vi "Virtual Labs 3.0.11.vi"() -> ()   [LabVIEW 2014]
panel:
  out "Actual volt":dbl
  out "Actual level":i32
  out "Ideal Vevel":i32
  out "Ideal voltage":dbl
  out "Stop":bool
  in  "Tab Control":T1(tab)
  in  "2":dbl(slide) scale=0.0..25.0
  out "?":dbl format="%#_3g"
  out "?":dbl format="%#_3g"
  out "?":dbl(slide) scale=0.0..684.0
  out "?":bool
  in  "Master Stop 2":bool
  out "Table 2":string[][](table)
  in  "Potentiometer\n       (4.7K)":dbl(knob) scale=0.0..4700.0 scale format="%#_6p"
  in  "Potentiometer (10K)":dbl(knob) scale=0.0..10000.0 scale format="%#_6p"
  out "?":dbl(slide) scale=0.0..684.0
  out "?":dbl format="%#_3g"
  out "?":dbl format="%#_3g"
  in  "?":dbl(slide)=25.0 scale=0.0..25.0
  out "?":bool
  in  "Master Stop":bool
  out "Table 3":string[][](table)
  out "Level Vs Output Voltage":cluster{"Y":dbl[], "Y":dbl[]}[](graph)
  out "Table 4":string[][](table)
  # "Manipal Institute of Technology  \n        Dept of Instrumentation and Control Engineering\n                                 V Sem (Instrumentation Lab)"
  # "VIRTUAL LABS"
  # "VIRTUAL LABS"
  # "EXPERIMENT NO.1"
  # "Liquid Level Measurement Using Capacitance Level Sensor\n\nObjective:  To design a signal conditioning circuit for measurement of liquid level using capacitance level sensors. \n\nApparatus required:\n\n            1\tCLS\n            2\tResistances\n            3\tAmplifier (741)\n            4\tDC power supply\n            5\tDMM"
  # "Ideal Case"
  # "Capacitive Level Sensor"
  # "Digital Multimeter"
  # "4-20m A"
  # "Level (in mm)"
  # "DC Voltage\n        (V)"
  # "Current (mA)"
  # "Animation Speed"
  # "Master Stop"
  # "Capacitive Level Sensor"
  # "Digital Multimeter"
  # "4-20m A"
  # "Level (in mm)"
  # "DC Voltage\n        (V)"
  # "Current (mA)"
  # "Animation Speed"
  # "Master Stop"
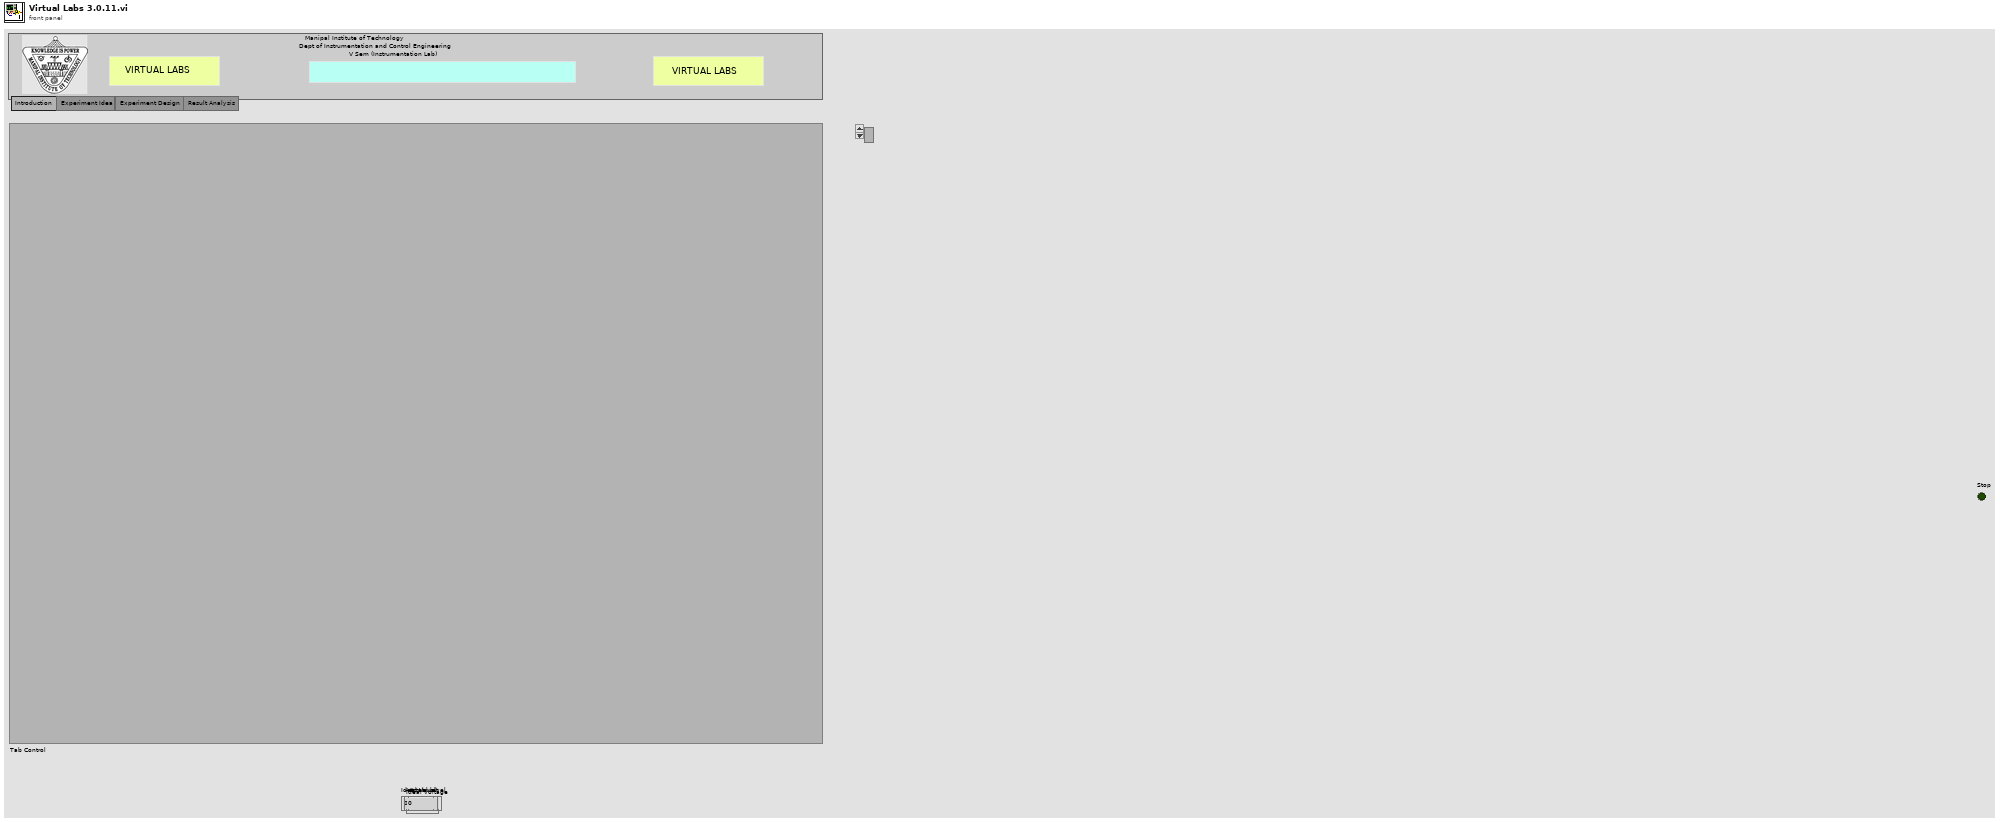
[diagram p1: front panel]
types:
  T1 = enum32{"Introduction", "Experiment Idea", "Experiment Design ", "Result Analysis"}
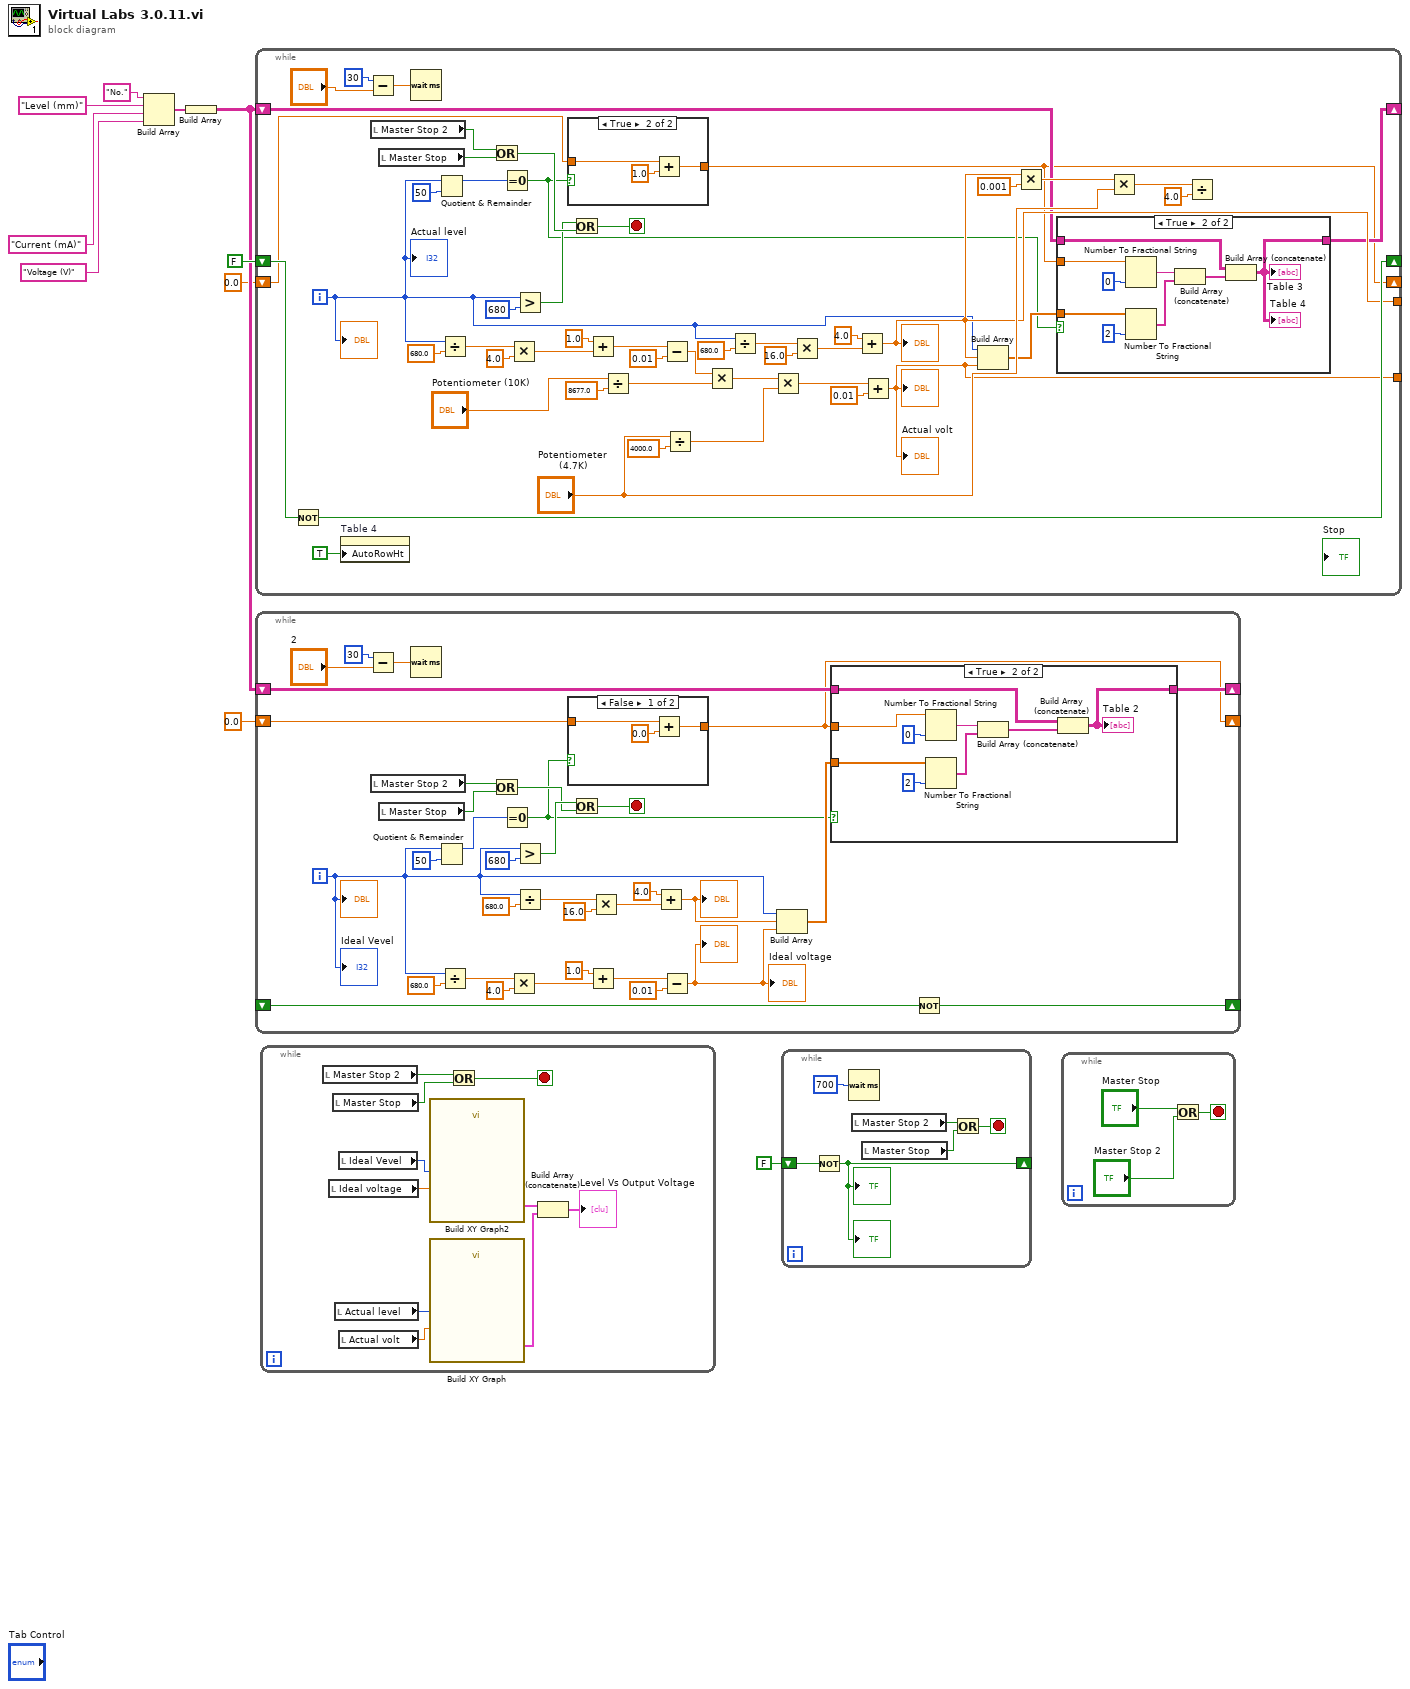
[diagram p0: block diagram]
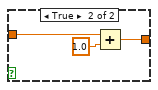
[diagram p2: hidden frame]
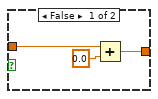
[diagram p4: hidden frame]
diagram:
  n1 = Build Array("No." ("element"), "Level (mm)" ("element"), "Current (mA)", "Voltage (V)") -> (w7:string[])
  n2 = Build Array(w7) -> (w6:string[][])
  n3 = while {
    shift-right: [w45] -> _
    shift-left: FALSE -> [w46]
    tunnel: [w14] -> _
    tunnel: [w25] -> _
    shift-right: [w24] -> _
    shift-left: w6 -> [w23]
    shift-right: [w11] -> _
    shift-left: 0.0 -> [w13]
    i -> [w15]
    stop <- w27 stop-if-true
    n4 = Not(x=w46) -> (.not. x?=w45:bool)
    n5 = property on="Table 4" class="Tbl (strict)"("AutoRowHt"=TRUE ("Autosizing Row Height")) -> ()  [unwired: 2 in, 2 out]
    n6 = Subtract(x=u32 30 ("milliseconds to wait"), y="?") -> (x-y=w34:dbl)
    n7 = local read "Master Stop 2"() -> (w21:bool)
    n8 = local read "Master Stop"() -> (w20:bool)
    n9 = Wait (ms)(milliseconds to wait=w34) -> ()  [unwired: 1 out]
    n10 = Quotient & Remainder(x=w15, y=50) -> (x-y*floor(x/y)=w16:i32)  [unwired: 1 out]
    n11 = Divide(x=w15, y=680.0) -> (x/y=w56:dbl)
    n12 = Or(x=w21, y=w20) -> (x .or. y?=w19:bool)
    n13 = Equal To 0?(x=w16) -> (x = 0?=w12:bool)
    n14 = Multiply(x=w56, y=4.0) -> (x*y=w54:dbl)
    n15 = Greater?(x=w15, y=680) -> (0:w18:bool)
    n16 = case shown="True" w12 {
      tunnel: w13 -> [w61 w65]
      tunnel: [w60 w64] -> w11
      frame False {
        n17 = Add(x=w61, y=0.0) -> (x+y=w60:dbl)
      }
      frame True {
        n18 = Add(x=w65, y=1.0) -> (x+y=w64:dbl)
      }
    }
    n19 = Or(x=w18, y=w19) -> (x .or. y?=w27:bool)
    n20 = Add(x=1.0, y=w54) -> (x+y=w48:dbl)
    n21 = Divide(x="Potentiometer (10K)", y=8677.0) -> (x/y=w38:dbl)
    n22 = Subtract(x=w48, y=0.01) -> (x-y=w37:dbl)
    n23 = Divide(x="Potentiometer\n       (4.7K)", y=4000.0) -> (x/y=w30:dbl)
    n24 = Multiply(x=w37, y=w38) -> (x*y=w31:dbl)
    n25 = Divide(x=w15, y=680.0) -> (x/y=w51:dbl)
    n26 = Multiply(x=w31, y=w30) -> (x*y=w29:dbl)
    n27 = Multiply(x=w51, y=16.0) -> (x*y=w53:dbl)
    n28 = Add(x=4.0, y=w53) -> (x+y=w25:dbl)
    "?" <- w25
    n29 = Add(x=w29, y=0.01) -> (x+y=w14:dbl)
    "?" <- w14
    "Actual volt" <- w14
    n30 = Build Array(w15, w25, w14) -> (w26:dbl[])
    n31 = Multiply(x=w25, y=0.001) -> (x*y=w43:dbl)
    n32 = case shown="True" w12 {
      tunnel: w26 -> [_ w75]
      tunnel: [w66 w67] -> w24
      tunnel: w23 -> [w66 w74]
      tunnel: w11 -> [_ w68]
      frame False {
      }
      frame True {
        n33 = Number To Fractional String(number=w68, precision (6)=i16 0) -> (F-format string=w71:string)  [unwired: 2 in]
        n34 = Number To Fractional String(number=w75, precision (6)=i16 2) -> (F-format string=w70:string[])  [unwired: 2 in]
        n35 = Build Array (concatenate)(w71, w70) -> (w69:string[])
        n36 = Build Array (concatenate)(w74, w69) -> (w67:string[][])
        "Table 3" <- w67
        "Table 4" <- w67
      }
    }
    n37 = Multiply(x=w43, y="Potentiometer\n       (4.7K)") -> (x*y=w42:dbl)
    n38 = Divide(x=w42, y=4.0) -> ()  [unwired: 1 out]
    "?" <- w15
    "Actual level" <- w15
  }
  n39 = while {
    shift-right: [w95] -> _
    shift-left: _ -> [w96]
    shift-right: [w86] -> _
    shift-left: w6 -> [w88]
    shift-right: [w76] -> _
    shift-left: 0.0 -> [w77]
    i -> [w83]
    stop <- w90 stop-if-true
    n40 = Subtract(x=u32 30 ("milliseconds to wait"), y="2") -> (x-y=w92:dbl)
    n41 = local read "Master Stop 2"() -> (w81:bool)
    n42 = local read "Master Stop"() -> (w80:bool)
    n43 = Wait (ms)(milliseconds to wait=w92) -> ()  [unwired: 1 out]
    n44 = Quotient & Remainder(x=w83, y=50) -> (x-y*floor(x/y)=w84:i32)  [unwired: 1 out]
    n45 = Divide(x=w83, y=680.0) -> (x/y=w106:dbl)
    n46 = Or(x=w81, y=w80) -> (x .or. y?=w79:bool)
    n47 = Equal To 0?(x=w84) -> (x = 0?=w78:bool)
    n48 = Multiply(x=w106, y=4.0) -> (x*y=w104:dbl)
    n49 = Greater?(x=w83, y=680) -> (0:w91:bool)
    n50 = Divide(x=w83, y=680.0) -> (x/y=w101:dbl)
    n51 = case shown="False" w78 {
      tunnel: w77 -> [w111 w115]
      tunnel: [w110 w114] -> w76
      frame False {
        n52 = Add(x=w111, y=0.0) -> (x+y=w110:dbl)
      }
      frame True {
        n53 = Add(x=w115, y=1.0) -> (x+y=w114:dbl)
      }
    }
    n54 = Or(x=w91, y=w79) -> (x .or. y?=w90:bool)
    n55 = Add(x=1.0, y=w104) -> (x+y=w98:dbl)
    n56 = Multiply(x=w101, y=16.0) -> (x*y=w103:dbl)
    n57 = Add(x=4.0, y=w103) -> (x+y=w87:dbl)
    "?" <- w87
    n58 = Subtract(x=w98, y=0.01) -> (x-y=w82:dbl)
    "?" <- w82
    "Ideal voltage" <- w82
    n59 = Build Array(w83, w87, w82) -> (w89:dbl[])
    n60 = case shown="True" w78 {
      tunnel: w89 -> [_ w125]
      tunnel: w88 -> [w116 w124]
      tunnel: [w116 w123] -> w86
      tunnel: w76 -> [_ w121]
      frame False {
      }
      frame True {
        n61 = Number To Fractional String(number=w121, precision (6)=i16 0) -> (F-format string=w119:string)  [unwired: 2 in]
        n62 = Number To Fractional String(number=w125, precision (6)=i16 2) -> (F-format string=w118:string[])  [unwired: 2 in]
        n63 = Build Array (concatenate)(w119, w118) -> (w117:string[])
        n64 = Build Array (concatenate)(w124, w117) -> (w123:string[][])
        "Table 2" <- w123
      }
    }
    n65 = Not(x=w96) -> (.not. x?=w95:bool)
    "?" <- w83
    "Ideal Vevel" <- w83
  }
  n66 = while {
    stop <- w127 stop-if-true
    n67 = local read "Master Stop 2"() -> (w128:bool)
    n68 = local read "Ideal voltage"() -> (w131:dbl)
    n69 = local read "Master Stop"() -> (w126:bool)
    n70 = local read "Actual level"() -> (w135:i32)
    n71 = local read "Ideal Vevel"() -> (w132:i32)
    n72 = local read "Actual volt"() -> (w134:dbl)
    n73 = call "Build XY Graph2"("Y Input"=w131, "X Input"=w132) -> ("XY Graph"=w130:cluster{"Y":dbl[], "Y":dbl[]}[])  [unwired: 3 in, 6 out]
    n74 = call "Build XY Graph"("Y Input"=w134, "X Input"=w135) -> ("XY Graph"=w133:cluster{"Y":dbl[], "Y":dbl[]}[])  [unwired: 3 in, 6 out]
    n75 = Or(x=w128, y=w126) -> (x .or. y?=w127:bool)
    n76 = Build Array (concatenate)(w130, w133) -> (→"Level Vs Output Voltage":cluster{"Y":dbl[], "Y":dbl[]}[])
  }
  n77 = while {
    shift-right: [w139] -> _
    shift-left: FALSE -> [w141]
    stop <- w136 stop-if-true
    n78 = Not(x=w141) -> (.not. x?=w139:bool)
    "?" <- w139
    "?" <- w139
    n79 = Wait (ms)(milliseconds to wait=u32 700) -> ()  [unwired: 1 out]
    n80 = local read "Master Stop 2"() -> (w138:bool)
    n81 = local read "Master Stop"() -> (w137:bool)
    n82 = Or(x=w138, y=w137) -> (x .or. y?=w136:bool)
  }
  n83 = while {
    stop <- w142 stop-if-true
    n84 = Or(x="Master Stop", y="Master Stop 2") -> (x .or. y?=w142:bool)
  }
